vi "Update Data(User Event).vi"(8 "error in (no error)":errorcluster, 10 "Data":cluster{"X":dbl[], "Y":dbl[]}[](array[cluster]), 11 "XYGraphOverview in":refnum<class "XYGraphOverview.lvclass">) -> (0 "error out":errorcluster, 3 "XYGraphOverview out":refnum<class "XYGraphOverview.lvclass">)   [LabVIEW 2020, in "XYGraphOverview.lvlib" / "XYGraphOverview.lvclass"]
uses:
  XYGraphOverview.lvclass
  XYGraphOverview.lvclass/XYGraphOverview.ctl
  <vilib>/Analysis/2dsp.llb/Decimate (single shot, DBL).vi
  Read Block Color.vi
  Read Sample Multiplier.vi
  <vilib>/Analysis/NI_AALPro.lvlib
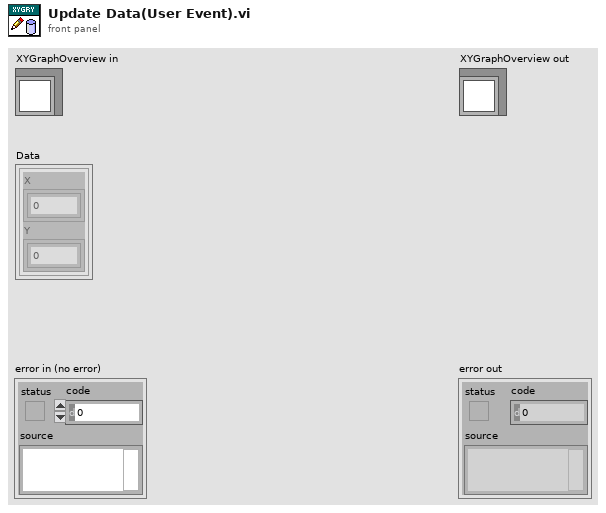
[diagram p1: front panel]
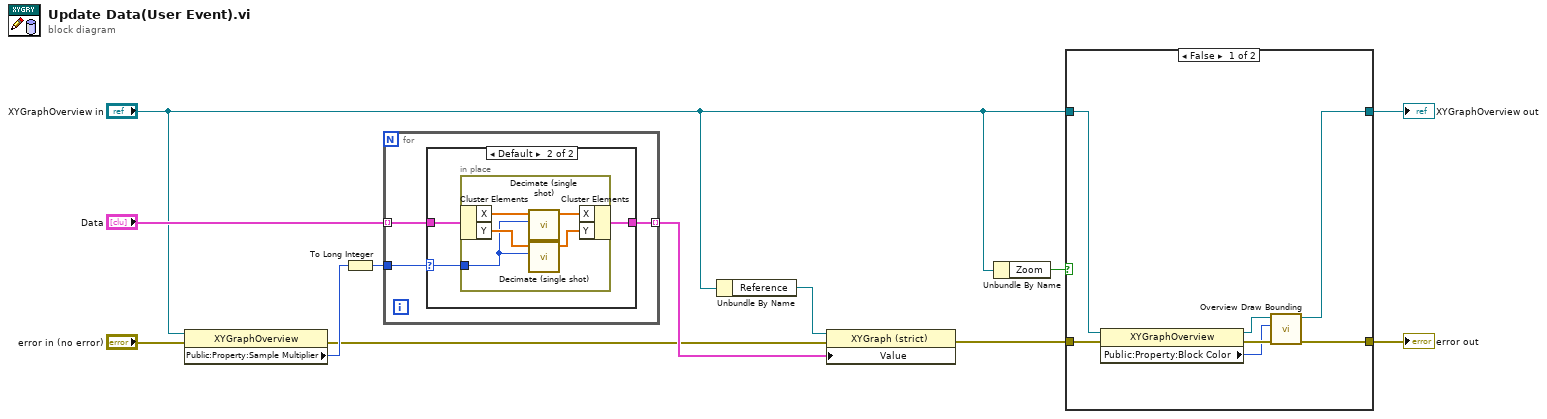
[diagram p0: block diagram]
diagram:
  n1 = property class="XYGraphOverview"(reference="XYGraphOverview in", error in="error in (no error)") -> (error out=w6:errorcluster, "Public:Property:Sample Multiplier"=w10:u32)  [unwired: 1 out]
  n2 = To Long Integer(number=w10) -> (32bit integer=w9:i32)
  n3 = for {
    tunnel: "Data" -> [w15] mode=indexing
    tunnel: w9 -> [w13]
    tunnel: [w14] -> w7 mode=indexing
    n4 = case shown="Default" w13 {
      selector: w13 -> [_ w17]
      tunnel: w15 -> [w16 w19]
      tunnel: [w16 w18] -> w14
      frame 0, 1 {
      }
      frame Default {
        n5 = in-place {
          in-place-border: w17 -> [w20]
          n6 = in-place-cluster #1(w19) -> ("X"=w23:dbl[], "Y"=w24:dbl[])
          n7 = call-poly <vilib>:"Decimate (single shot).vi"("decimating factor"=w20, "X"=w23) -> ("Decimated Array"=w22:dbl[])  [unwired: 8 in, 1 out]
          n8 = call-poly <vilib>:"Decimate (single shot).vi"("decimating factor"=w20, "X"=w24) -> ("Decimated Array"=w21:dbl[])  [unwired: 8 in, 1 out]
          n9 = in-place-cluster #1("X"=w22, "Y"=w21) -> (w18:cluster{"X":dbl[], "Y":dbl[]})
        }
      }
    }
  }
  n10 = Unbundle By Name("XYGraphOverview in") -> ("Reference"=w8:refnum<vi>)
  n11 = property class="XYGraph (strict)"(reference=w8, error in=w6, "Value"=w7) -> (error out=w4:errorcluster)  [unwired: 1 out]
  n12 = Unbundle By Name("XYGraphOverview in") -> ("Zoom"=w5:bool)
  n13 = case shown="False" w5 {
    tunnel: w4 -> [w28 w32]
    tunnel: "XYGraphOverview in" -> [w27 w33]
    tunnel: [w25 w33] -> w2
    tunnel: [w26 w32] -> w1
    frame False {
      n14 = property class="XYGraphOverview"(reference=w27, error in=w28) -> (reference out=w30:refnum<class "XYGraphOverview.lvclass">, error out=w31:errorcluster, "Public:Property:Block Color"=w29:u32)
      n15 = call "Overview Draw Bounding.vi"("error in (no error)"=w31, "Color"=w29, "XYGraphOverview in"=w30) -> ("error out"=w26:errorcluster, "XYGraphOverview out"=w25:refnum<class "XYGraphOverview.lvclass">)  [unwired: 7 in]
    }
    frame True {
    }
  }
  "error out" <- w1
  "XYGraphOverview out" <- w2
